vi "climbLoop.vi"() -> ()   [LabVIEW 2018]
uses:
  climbSMEnum.ctl
  climbStateEnum.ctl
  climbPlatformEnum.ctl
  climbStilt/climbStiltStateEnum.ctl
  driveClimbStateEnum.ctl
  <userlib>/836-Library/System/TDMS_V2/Support/TDMS_DevRef.ctl
  <userlib>/836-Library/System/TDMS_V2/Support/Logging_Settings.ctl
  <userlib>/836-Library/System/TDMS_V2/Support/Group_FIFO_Config.ctl
  <userlib>/836-Library/System/TDMS_V2/Support/Channel_FIFO_Config.ctl
panel:
  in  "Drive Enc Trig Point L2":dbl=-35.0
  out "timed out?":bool=TRUE
  in  "Drive Enc Trig Point L3":dbl=-35.0
  in  "Drive Speed":dbl=-0.2
  in  "Encoder Trigger Point":dbl=-12.9
  out "Waveform Chart":u16(graph)=12
  out "driveAvgPos(inch)":dbl=-5.765416124131944
  in  "Little wheel abs Power First 2":dbl=0.9
  in  "Wait to Extend (ms)":u32=500
  in  "Little wheel abs Power First":dbl=0.6
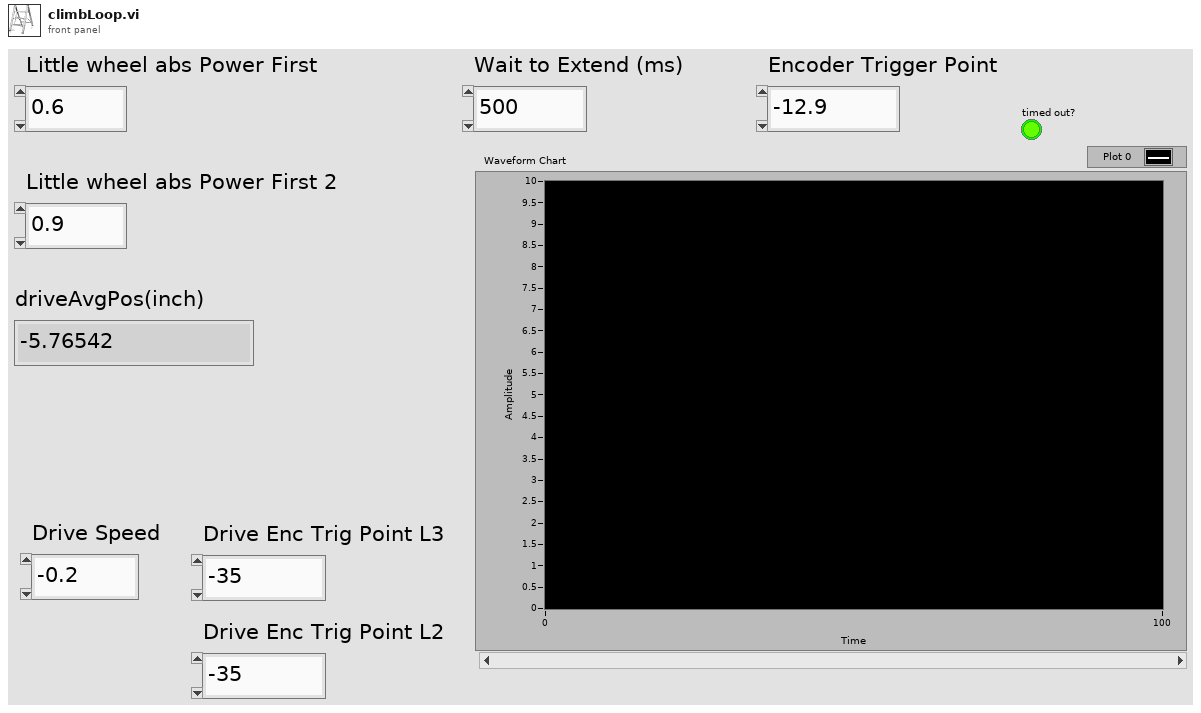
[diagram p1: front panel]
types:
  T1 = typedef "climbStateEnum.ctl" = enum16{"doNothing", "Auto Mode", "Safely Lower", "Test Mode"}
  T2 = typedef "climbSMEnum.ctl" = enum16{"1 - do nothing", "2 - Prep Systems", "3 - small startz", "4 - lift stiltz", "5 - drive little wheel 1", "6 - retract front stilt", "7 - drive little wheel 2", "8 - retract rear stilt", "9 - drive to middle", "10 - STOP", "7b - L2-L3 Drive Little Wheel 2", "8b - Balance", "10b - Balance Drive"}
  T3 = typedef "WPI_MotorControlDeviceRef.ctl" = cluster{"DeviceStatus":errorcluster, "Type":T4, "PWM":cluster{"PWM Channel":T5, "DeadBand":T6}, "CAN":cluster{"Device Number":u8, "SetOutput VI Ref":variant, "GetOutput VI Ref":variant, "Enable VI Ref":variant, "Disable VI Ref":variant, "Data":variant}, "Invert":bool, "DIO PWM":cluster{"PWM \"Enable\" Channel":T5, "DIOChannel":T7, "PWM Rate":dbl}}
  T4 = typedef "WPI_MotorControlType.ctl" = enum16{"PWM", "CAN", "DIO PWM"}
  T5 = typedef "FPGA_DIOPWMChannel.ctl" = enum8{"PWM 0", "PWM 1", "PWM 2", "PWM 3", "PWM 4", "PWM 5", "PWM 6", "PWM 7", "PWM 8", "PWM 9", "PWM MXP 0", "PWM MXP 1", "PWM MXP 2", "PWM MXP 3", "PWM MXP 4", "PWM MXP 5", "PWM MXP 6", "PWM MXP 7", "PWM MXP 8", "PWM MXP 9", "Invalid"}
  T6 = typedef "WPI_PWMDeadband.ctl" = cluster{"Name":string, "maxPositivePwm":i32, "minPositivePwm":i32, "centerPwm":i32, "maxNegativePwm":i32, "minNegativePwm":i32, "angularRange":u16}
  T7 = typedef "FPGA_DIOChannel.ctl" = enum8{"DIO 0", "DIO 1", "DIO 2", "DIO 3", "DIO 4", "DIO 5", "DIO 6", "DIO 7", "DIO 8", "DIO 9", "DIO MXP 0", "DIO MXP 1", "DIO MXP 2", "DIO MXP 3", "DIO MXP 4", "DIO MXP 5", "DIO MXP 6", "DIO MXP 7", "DIO MXP 8", "DIO MXP 9", "DIO MXP 10", "DIO MXP 11", "DIO MXP 12", "DIO MXP 13", "DIO MXP 14", "DIO MXP 15", "SPI Port CS1", "SPI Port CS2", "SPI Port CS3", "SPI Port MISO", "SPI Port MOSI", "Invalid"}
  T8 = typedef "WPI_DigitalInputDevRef.ctl" = cluster{"DevStatus":errorcluster, "DIO Channel":T7}
  T9 = typedef "WPI_SolenoidDevRef.ctl" = cluster{"DevStatus":errorcluster, "Pneumatics Control Module":u8, "Forward Solenoid Channel":T10, "Reverse Solenoid Channel":T10}
  T10 = typedef "WPI_SolenoidChannel.ctl" = enum8{"Solenoid 0", "Solenoid 1", "Solenoid 2", "Solenoid 3", "Solenoid 4", "Solenoid 5", "Solenoid 6", "Solenoid 7", "Invalid"}
  T11 = enum16{"L1 -> L3 Platform", "L1 -> L2 Platform", "L2 -> L3 Platform", "No Climb"}
  T12 = enum16{"Both Locked", "Skid Unlock/Powered Locked", "Skid Locked/Powered Unlocked", "Both Unlocked"}
  T13 = typedef "climbPlatformEnum.ctl" = enum16{"L1 -> L3 Platform", "L1 -> L2 Platform", "L2 -> L3 Platform", "No Climb"}
  T14 = typedef "driveClimbStateEnum.ctl" = enum16{"Do Nothing", "Drive Forward", "Slow Manual Drive"}
  T15 = typedef "climbStiltStateEnum.ctl" = enum16{"doNothing", "Start/Safely Lower Both", "Both Extend", "Front Retract", "Both Retract", "Test Mode", "Balance"}
  T16 = typedef "TDMS_DevRef.ctl" = cluster{"Name":string, "File Ref":refnum<k34>, "Start Time":timestamp, "Logging Settings":T17, "Group FIFO Config":T18[], "Data To Write":refnum<data-value>, "semaphore":T20, "Ref Time Reset":refnum<k4>}
  T17 = typedef "Logging_Settings.ctl" = cluster{"Data Grab Period":dbl, "File Write Period":dbl, "Max Stored Size":dbl, "Burst Size":dbl}
  T18 = typedef "Group_FIFO_Config.ctl" = cluster{"Group":string, "Channels":T19[], "Channel Names":string[]}
  T19 = typedef "Channel_FIFO_Config.ctl" = cluster{"Channel":string, "FIFO":refnum<k33>}
  T20 = typedef "Semaphore RefNum" = refnum<k1>
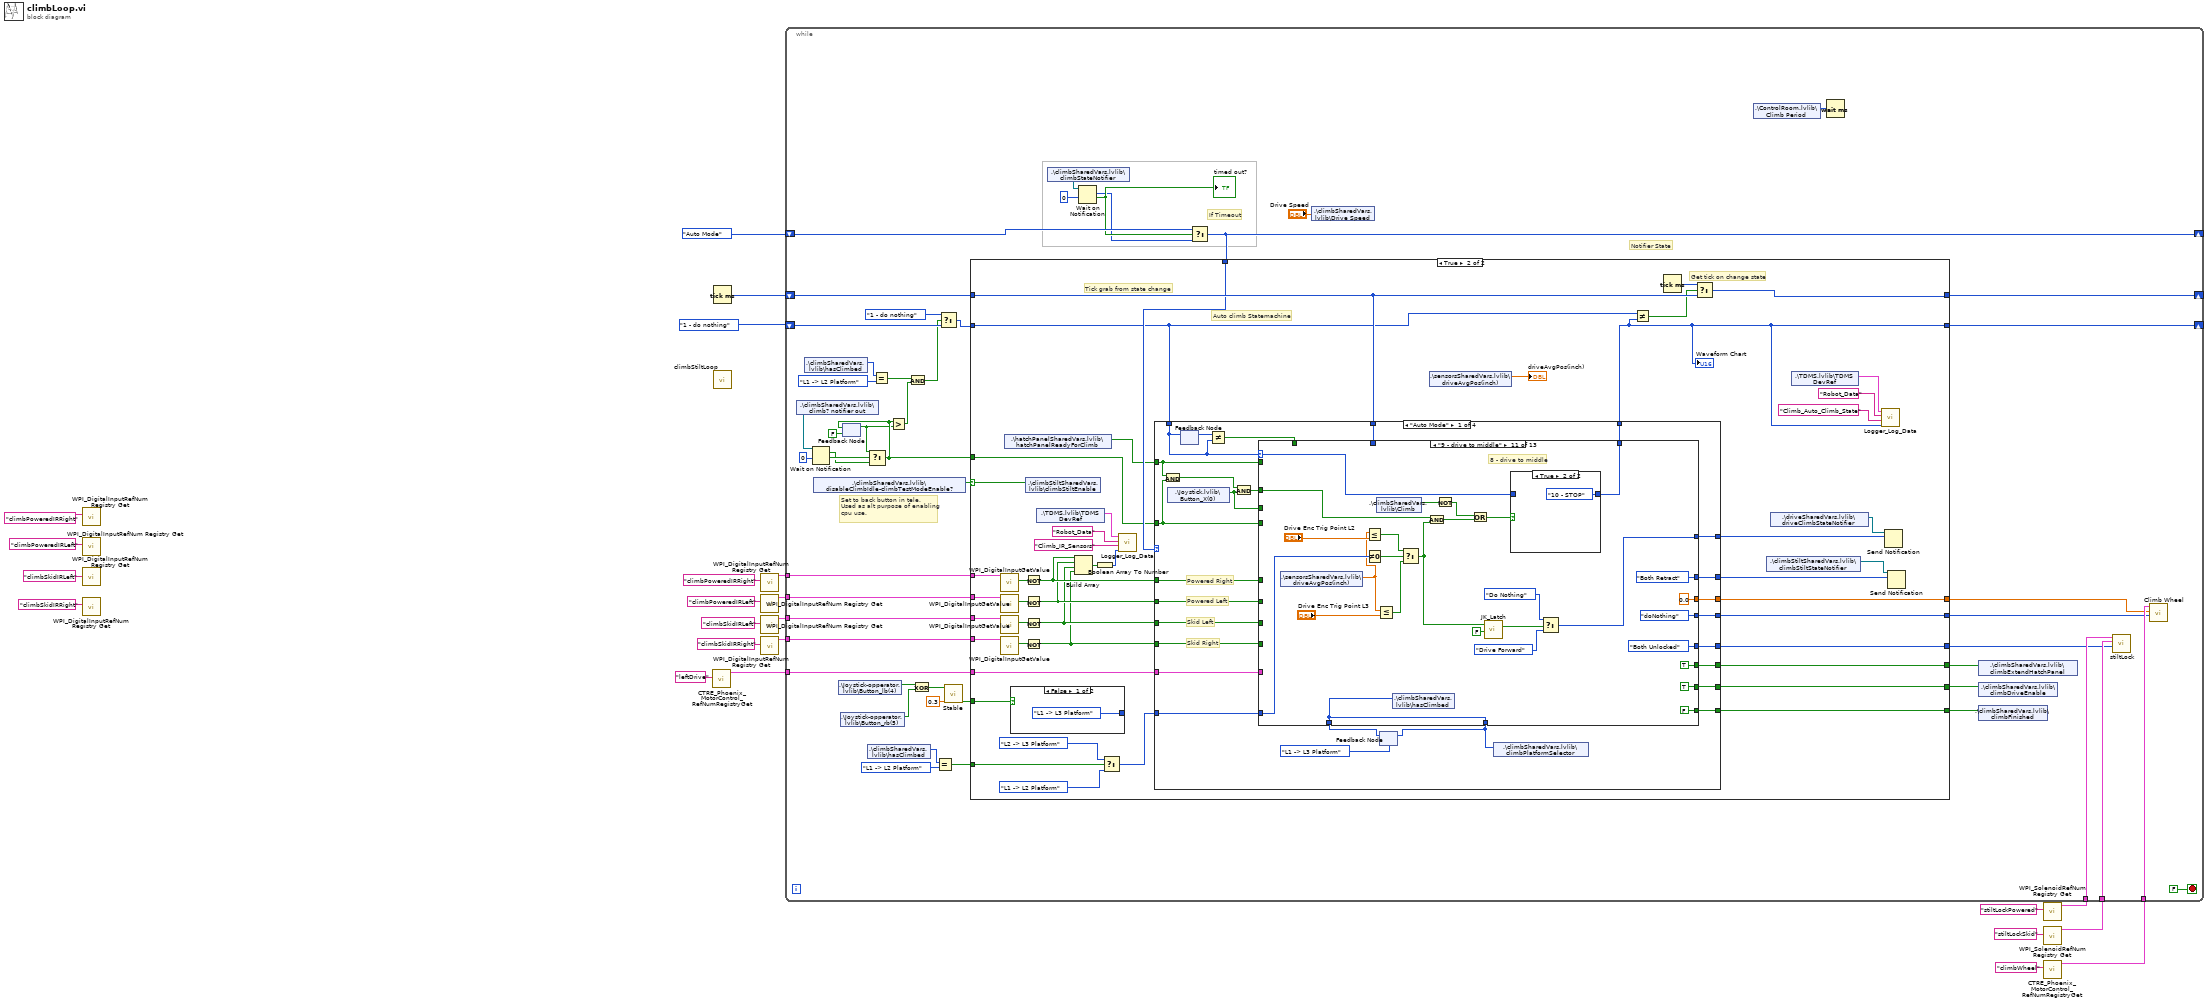
[diagram p0: block diagram]
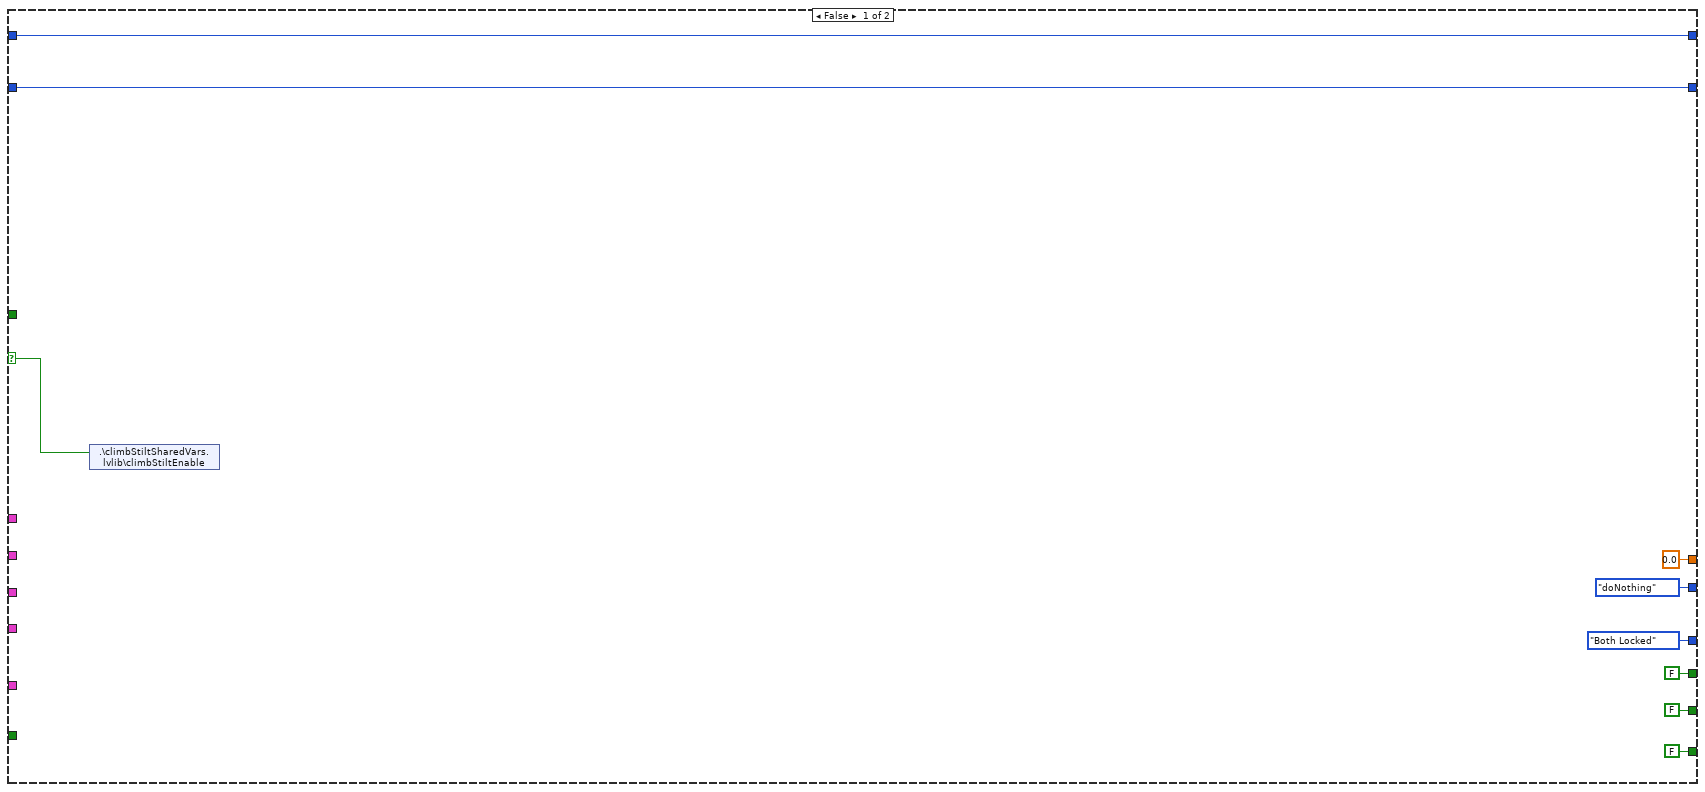
[diagram p2: hidden frame]
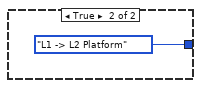
[diagram p3: hidden frame]
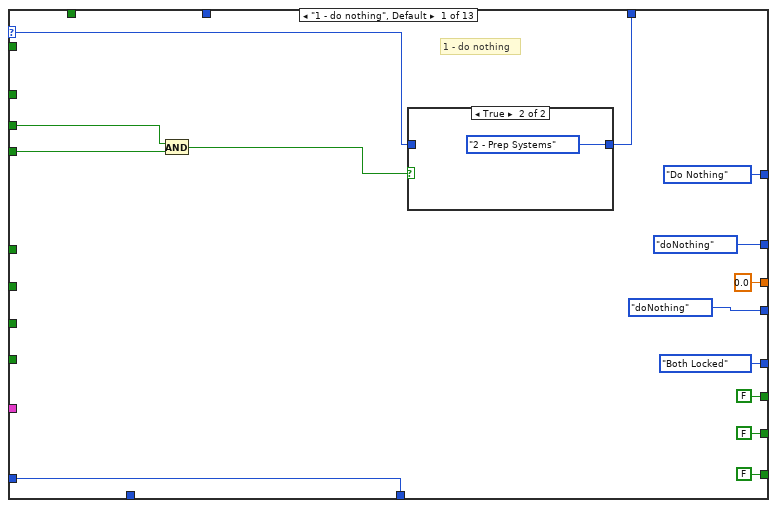
[diagram p4: hidden frame]
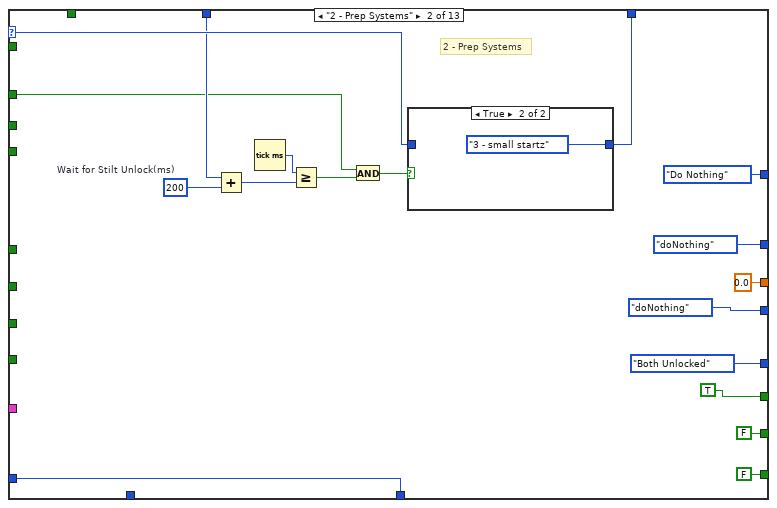
[diagram p6: hidden frame]
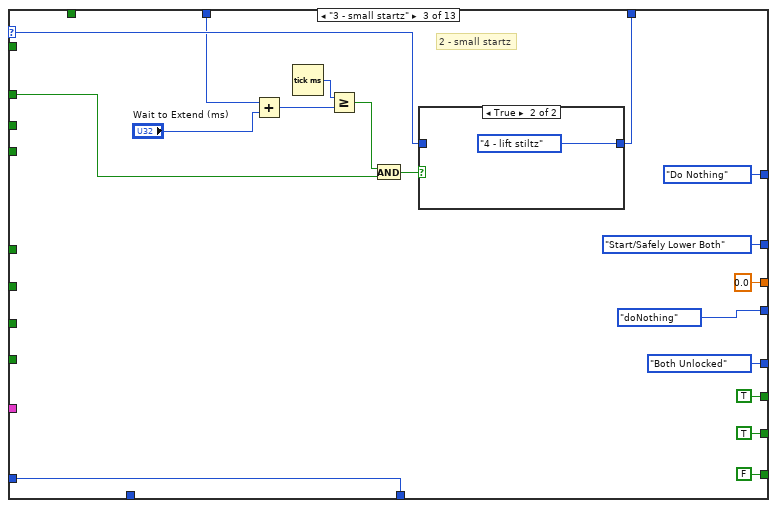
[diagram p8: hidden frame]
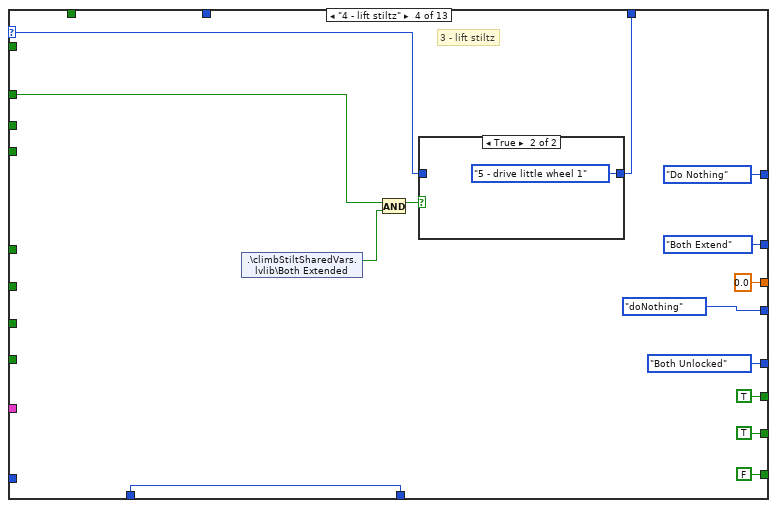
[diagram p10: hidden frame]
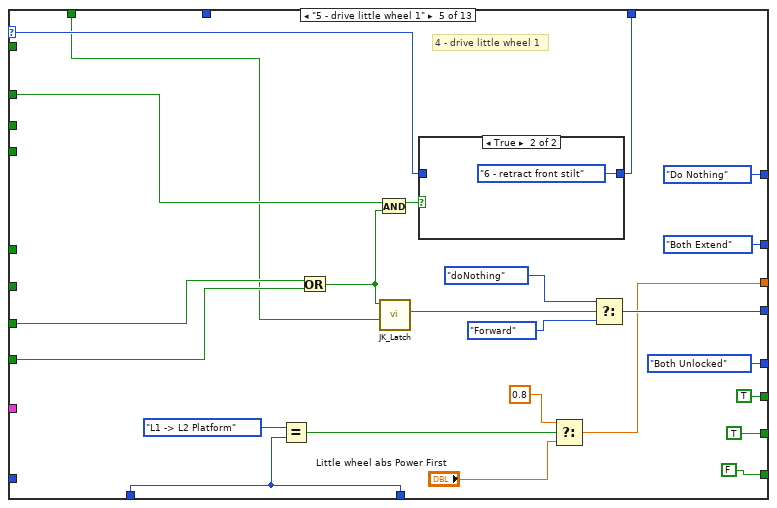
[diagram p12: hidden frame]
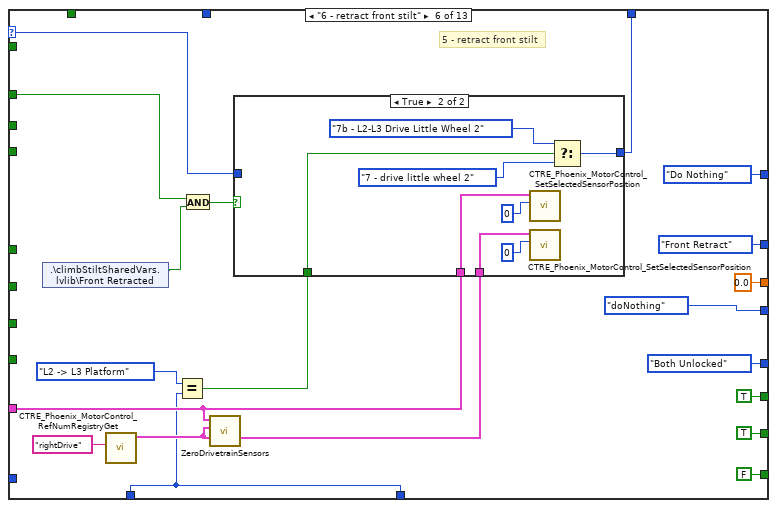
[diagram p14: hidden frame]
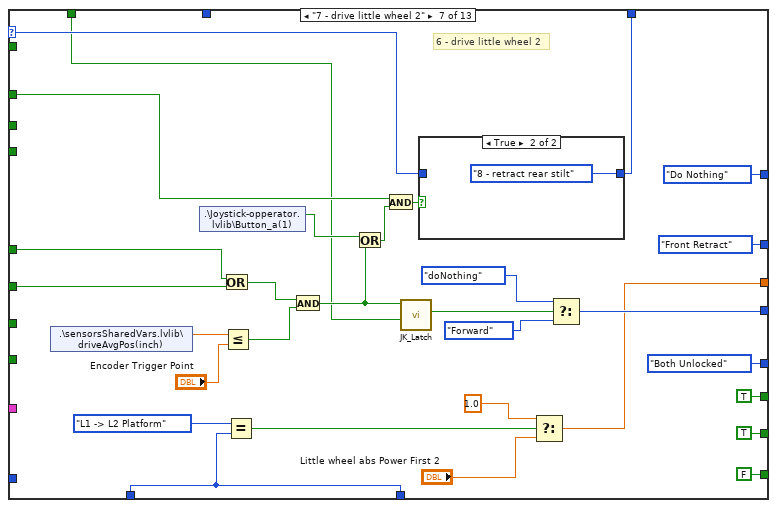
[diagram p16: hidden frame]
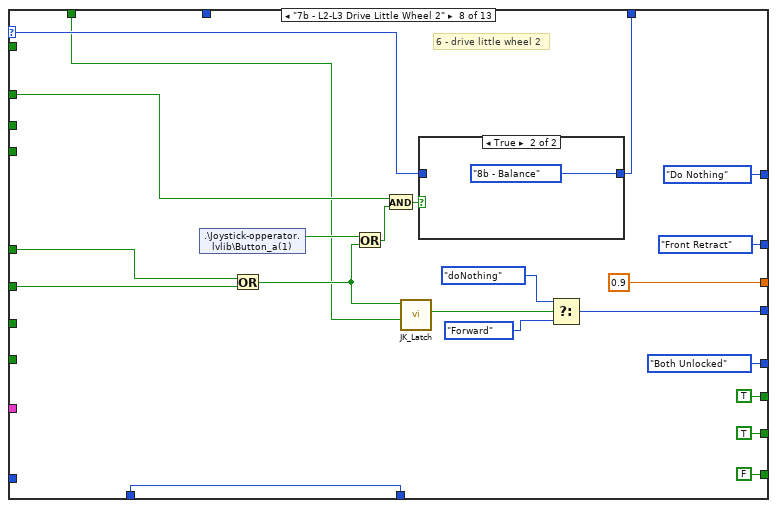
[diagram p18: hidden frame]
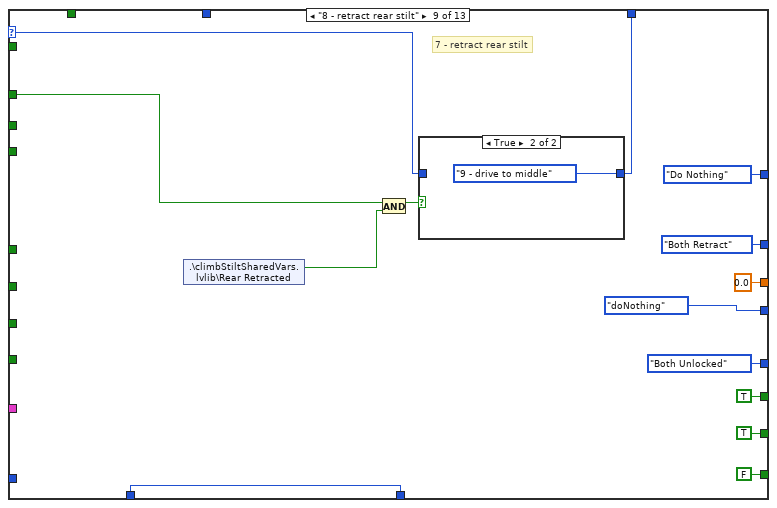
[diagram p20: hidden frame]
diagram:
  n1 = call <vilib>:"WPI_DigitalInputRefNum Registry Get.vi"("refnum name"="climbPoweredIRRight") -> ()  [unwired: 9 in, 2 out]
  n2 = call <vilib>:"WPI_DigitalInputRefNum Registry Get.vi"("refnum name"="climbPoweredIRLeft") -> ()  [unwired: 9 in, 2 out]
  n3 = call <vilib>:"WPI_DigitalInputRefNum Registry Get.vi"("refnum name"="climbSkidIRLeft") -> ()  [unwired: 9 in, 2 out]
  n4 = call <vilib>:"WPI_DigitalInputRefNum Registry Get.vi"("refnum name"="climbSkidIRRight") -> ()  [unwired: 9 in, 2 out]
  n5 = call <vilib>:"CTRE_Phoenix_MotorControl_RefNumRegistryGet.vi"("refnum name"="leftDrive") -> ("PhoenixMotorControlDevRef"=w21:T3)  [unwired: 9 in, 1 out]
  n6 = Tick Count (ms)() -> (millisecond timer value=w23:u32)
  n7 = call "climbStiltLoop.vi"() -> ()  [unwired: 12 in]
  n8 = call <vilib>:"WPI_DigitalInputRefNum Registry Get.vi"("refnum name"="climbPoweredIRRight") -> ("DigitalInputDevRef"=w1:T8)  [unwired: 9 in, 1 out]
  n9 = call <vilib>:"WPI_DigitalInputRefNum Registry Get.vi"("refnum name"="climbPoweredIRLeft") -> ("DigitalInputDevRef"=w2:T8)  [unwired: 9 in, 1 out]
  n10 = call <vilib>:"WPI_DigitalInputRefNum Registry Get.vi"("refnum name"="climbSkidIRLeft") -> ("DigitalInputDevRef"=w3:T8)  [unwired: 9 in, 1 out]
  n11 = call <vilib>:"WPI_DigitalInputRefNum Registry Get.vi"("refnum name"="climbSkidIRRight") -> ("DigitalInputDevRef"=w4:T8)  [unwired: 9 in, 1 out]
  n12 = call <vilib>:"WPI_SolenoidRefNum Registry Get.vi"("refnum name"="stiltLockPowered") -> ("SolenoidDevRef"=w18:T9)  [unwired: 9 in, 1 out]
  n13 = call <vilib>:"WPI_SolenoidRefNum Registry Get.vi"("refnum name"="stiltLockSkid") -> ("SolenoidDevRef"=w17:T9)  [unwired: 9 in, 1 out]
  n14 = call <vilib>:"CTRE_Phoenix_MotorControl_RefNumRegistryGet.vi"("refnum name"="climbWheel") -> ("PhoenixMotorControlDevRef"=w14:T3)  [unwired: 9 in, 1 out]
  n15 = while {
    shift-right: [w70] -> _
    shift-left: climbStateEnum."Auto Mode" ("Climb State") -> [w68]
    shift-right: [w69] -> _
    shift-left: climbSMEnum."1 - do nothing" ("Climb SM") -> [w29]
    shift-right: [w73] -> _
    shift-left: w23 -> [w72]
    tunnel: w21 -> [w71]
    tunnel: w18 -> [w67]
    tunnel: w17 -> [w66]
    tunnel: w14 -> [w65]
    tunnel: w4 -> [w42]
    tunnel: w3 -> [w41]
    tunnel: w2 -> [w40]
    tunnel: w1 -> [w39]
    stop <- FALSE stop-if-true
    # "Set to back button in tele.\nUsed as alt purpose of enabling\ncpu use."
    # "Notifier State"
    # "If Timeout"
    n16 = shared-variable ".\\climbSharedVars.lvlib\\climb? notifier out"() -> (w51:refnum<notifier>)  [unwired: 1 in, 1 out]
    n17 = shared-variable ".\\climbSharedVars.lvlib\\hasClimbed"() -> (w36:T11)  [unwired: 1 in, 1 out]
    n18 = Wait on Notification(notifier=w51, timeout in ms (-1)=0) -> (notification=w52:bool, timed out?=w53:bool)  [unwired: 2 in, 2 out]
    n19 = shared-variable ".\\climbSharedVars.lvlib\\disableClimbIdle-climbTestModeEnable?"() -> (w48:bool)  [unwired: 1 in, 1 out]
    n20 = shared-variable ".\\Joystick-opperator.lvlib\\Button_lb(4)"() -> (w47:bool)  [unwired: 1 in, 1 out]
    n21 = shared-variable ".\\Joystick-opperator.lvlib\\Button_rb(5)"() -> (w46:bool)  [unwired: 1 in, 1 out]
    n22 = feedback #1(FALSE ("create if not found? (T)")) -> (w33:bool)
    n23 = shared-variable ".\\climbSharedVars.lvlib\\hasClimbed"() -> (w26:T11)  [unwired: 1 in, 1 out]
    n24 = Select(t=w33, s=w53, f=w52) -> (s? t:f=w34:bool)
    n25 = feedback-in #1(w34) -> ()
    n26 = Equal?(x=w36, y=T11."L1 -> L2 Platform") -> (x = y?=w31:bool)
    n27 = Greater?(x=w34, y=w33) -> (0:w32:bool)
    n28 = And(x=w31, y=w32) -> (x .and. y?=w28:bool)
    n29 = Exclusive Or(1:w46, 2:w47) -> (0:w45:bool)
    n30 = Equal?(x=w26, y=T11."L1 -> L2 Platform") -> (x = y?=w24:bool)
    n31 = Select(t=climbSMEnum."1 - do nothing", s=w28, f=w29) -> (s? t:f=w27:T2)
    n32 = call <userlib>:"Stable.vi"("Eval Period (sec)"=0.3, "Signal Input"=w45) -> ("Stable"=w44:bool)  [unwired: 9 in]
    n33 = shared-variable ".\\climbSharedVars.lvlib\\climbStateNotifier"() -> (w61:refnum<notifier>)  [unwired: 1 in, 1 out]
    n34 = Wait on Notification(notifier=w61, timeout in ms (-1)=0) -> (notification=w58:T1, timed out?=w62:bool)  [unwired: 2 in, 2 out]
    "timed out?" <- w62
    n35 = Select(t=w68, s=w62, f=w58) -> (s? t:f=w70:T1)
    n36 = case shown="True" w48 {
      selector: w48 -> [w75 w109]
      tunnel: [w76 w129] -> w73
      tunnel: w72 -> [w76 w128]
      tunnel: w71 -> [_ w127]
      tunnel: w70 -> [_ w126]
      tunnel: [w74 w125] -> w69
      tunnel: [enum16{"doNothing", "Forward", "Backward"}."doNothing" ("Enum") w124] -> w64
      tunnel: [0.0 ("Little wheel abs Power First 2") w119] -> w60
      tunnel: [FALSE w114] -> w57
      tunnel: [FALSE w113] -> w56
      tunnel: [FALSE w112] -> w55
      tunnel: [T12."Both Locked" ("Lock State") w111] -> w54
      tunnel: w34 -> [_ w110]
      tunnel: w44 -> [_ w105]
      tunnel: w42 -> [_ w100]
      tunnel: w41 -> [_ w99]
      tunnel: w40 -> [_ w98]
      tunnel: w39 -> [_ w97]
      tunnel: w27 -> [w74 w87]
      tunnel: w24 -> [_ w83]
      frame False {
        n37 = shared-variable ".\\climbStiltSharedVars.lvlib\\climbStiltEnable"(w75) -> ()  [unwired: 1 in, 1 out]
      }
      frame True {
        # "Auto climb Statemachine"
        # "Tick grab from state change"
        # "Get tick on change state"
        n38 = call <vilib>:"WPI_DigitalInputGetValue.vi"("DigitalInputDevRef"=w97) -> ("Value"=w101:bool)  [unwired: 8 in, 2 out]
        n39 = call <vilib>:"WPI_DigitalInputGetValue.vi"("DigitalInputDevRef"=w98) -> ("Value"=w102:bool)  [unwired: 8 in, 2 out]
        n40 = call <vilib>:"WPI_DigitalInputGetValue.vi"("DigitalInputDevRef"=w99) -> ("Value"=w103:bool)  [unwired: 8 in, 2 out]
        n41 = call <vilib>:"WPI_DigitalInputGetValue.vi"("DigitalInputDevRef"=w100) -> ("Value"=w104:bool)  [unwired: 8 in, 2 out]
        n42 = shared-variable ".\\hatchPanelSharedVars.lvlib\\hatchPanelReadyForClimb"() -> (w115:bool)  [unwired: 1 in, 1 out]
        n43 = case shown="False" w105 {
          tunnel: [climbPlatformEnum."L1 -> L3 Platform" ("climbPlatformSelector") climbPlatformEnum."L1 -> L2 Platform" ("climbPlatformSelector")] -> _
          frame False {
          }
          frame True {
          }
        }
        n44 = Not(x=w101) -> (.not. x?=w91:bool)
        n45 = Not(x=w102) -> (.not. x?=w90:bool)
        n46 = Not(x=w103) -> (.not. x?=w89:bool)
        n47 = Not(x=w104) -> (.not. x?=w88:bool)
        n48 = shared-variable ".\\climbStiltSharedVars.lvlib\\climbStiltEnable"(w109) -> ()  [unwired: 1 in, 1 out]
        n49 = shared-variable ".\\TDMS.lvlib\\TDMS DevRef"() -> (w95:T16)  [unwired: 1 in, 1 out]
        n50 = Build Array(w91, w90, w89, w88) -> (w92:bool[])
        n51 = Boolean Array To Number(Boolean array=w92) -> (number=w96:u32)
        n52 = Select(t=climbPlatformEnum."L2 -> L3 Platform" ("climbPlatformSelector"), s=w83, f=climbPlatformEnum."L1 -> L2 Platform" ("climbPlatformSelector")) -> (s? t:f=w85:T13)
        n53 = call <userlib>:"Logger_Log_Data.vi"("Data"=w96, "Channel"="Climb_IR_Sensors", "Group"="Robot_Data", "TDMS DevRef"=w95) -> ()  [unwired: 7 in, 1 out]
        n54 = case shown="\"Auto Mode\"" w126 {
          tunnel: [w158 enum16{"doNothing", "Forward", "Backward"}."doNothing" ("Enum") enum16{"doNothing", "Forward", "Backward"}."doNothing" ("Enum") enum16{"doNothing", "Forward", "Backward"}."doNothing" ("Enum")] -> w124
          tunnel: w87 -> [w133 _ _ _]
          tunnel: [w157 climbStiltStateEnum."Start/Safely Lower Both" ("notification") w440 climbStiltStateEnum."doNothing" ("notification")] -> w122
          tunnel: [w156 climbSMEnum."1 - do nothing" ("Climb SM") climbSMEnum."1 - do nothing" ("Climb SM") climbSMEnum."1 - do nothing" ("Climb SM")] -> w125
          tunnel: w128 -> [w155 _ _ _]
          tunnel: [w154 0.0 ("Little wheel abs Power First 2") 0.0 ("Little wheel abs Power First 2") 0.0 ("Little wheel abs Power First 2")] -> w119
          tunnel: w127 -> [w153 _ _ _]
          tunnel: [w152 driveClimbStateEnum."Do Nothing" ("notification") driveClimbStateEnum."Do Nothing" ("notification") driveClimbStateEnum."Do Nothing" ("notification")] -> w116
          tunnel: w110 -> [w148 _ _ _]
          tunnel: [w151 T12."Both Unlocked" ("Lock State") T12."Both Unlocked" ("Lock State") T12."Both Locked" ("Lock State")] -> w111
          tunnel: [w150 TRUE TRUE FALSE] -> w113
          tunnel: w115 -> [w149 _ w437 _]
          tunnel: [w147 TRUE TRUE FALSE] -> w114
          tunnel: [w146 FALSE FALSE FALSE] -> w112
          tunnel: w85 -> [w145 _ _ _]
          tunnel: w88 -> [w141 _ _ _]
          tunnel: w89 -> [w140 _ _ _]
          tunnel: w90 -> [w139 _ _ _]
          tunnel: w91 -> [w138 _ _ _]
          frame "Auto Mode" {
            # "Skid Right"
            # "Skid Left"
            # "Powered Left"
            # "Powered Right"
            n55 = And(x=w149, y=w148) -> (x .and. y?=w137:bool)
            n56 = shared-variable ".\\Joystick.lvlib\\Button_X(0)"() -> (w135:bool)  [unwired: 1 in, 1 out]
            n57 = feedback-in #2(w133) -> ()
            n58 = feedback #2() -> (w134:T2)  [unwired: 1 in]
            n59 = Not Equal?(x=w134, y=w133) -> (x != y?=w132:bool)
            n60 = And(x=w137, y=w135) -> (x .and. y?=w136:bool)
            n61 = feedback #3(climbPlatformEnum."L1 -> L3 Platform" ("climbPlatformSelector")) -> (w143:T13)
            n62 = case shown="\"9 - drive to middle\"" w133 {
              selector: w133 -> [w169 w189 w209 w228 w254 w275 w314 w338 w354 w374 w394 w414 w424]
              tunnel: [enum16{"doNothing", "Forward", "Backward"}."doNothing" ("Enum") enum16{"doNothing", "Forward", "Backward"}."doNothing" ("Enum") enum16{"doNothing", "Forward", "Backward"}."doNothing" ("Enum") enum16{"doNothing", "Forward", "Backward"}."doNothing" ("Enum") w248 enum16{"doNothing", "Forward", "Backward"}."doNothing" ("Enum") w309 w333 enum16{"doNothing", "Forward", "Backward"}."doNothing" ("Enum") enum16{"doNothing", "Forward", "Backward"}."doNothing" ("Enum") enum16{"doNothing", "Forward", "Backward"}."doNothing" ("Enum") enum16{"doNothing", "Forward", "Backward"}."doNothing" ("Enum") enum16{"doNothing", "Forward", "Backward"}."doNothing" ("Enum")] -> w158
              tunnel: [climbStiltStateEnum."doNothing" ("notification") climbStiltStateEnum."doNothing" ("notification") climbStiltStateEnum."Start/Safely Lower Both" ("notification") climbStiltStateEnum."Both Extend" ("notification") climbStiltStateEnum."Both Extend" ("notification") climbStiltStateEnum."Front Retract" ("notification") climbStiltStateEnum."Front Retract" ("notification") climbStiltStateEnum."Front Retract" ("notification") climbStiltStateEnum."Both Retract" ("notification") climbStiltStateEnum."Balance" ("notification") climbStiltStateEnum."Both Retract" ("notification") climbStiltStateEnum."doNothing" ("notification") climbStiltStateEnum."doNothing" ("notification")] -> w157
              tunnel: [w170 w190 w210 w227 w253 w274 w313 w337 w353 w373 w393 w414 w424] -> w156
              tunnel: w155 -> [_ w180 w204 _ _ _ _ _ _ w357 _ _ _]
              tunnel: [0.0 ("Little wheel abs Power First 2") 0.0 ("Little wheel abs Power First 2") 0.0 ("Little wheel abs Power First 2") 0.0 ("Little wheel abs Power First 2") w236 0.0 ("Little wheel abs Power First 2") w290 0.9 ("t") 0.0 ("Little wheel abs Power First 2") 0.0 ("Little wheel abs Power First 2") 0.0 ("Little wheel abs Power First 2") 0.0 ("Little wheel abs Power First 2") 0.0 ("Little wheel abs Power First 2")] -> w154
              tunnel: w153 -> [_ _ _ _ _ w262 _ _ _ _ _ _ _]
              tunnel: [driveClimbStateEnum."Do Nothing" ("notification") driveClimbStateEnum."Do Nothing" ("notification") driveClimbStateEnum."Do Nothing" ("notification") driveClimbStateEnum."Do Nothing" ("notification") driveClimbStateEnum."Do Nothing" ("notification") driveClimbStateEnum."Do Nothing" ("notification") driveClimbStateEnum."Do Nothing" ("notification") driveClimbStateEnum."Do Nothing" ("notification") driveClimbStateEnum."Do Nothing" ("notification") driveClimbStateEnum."Do Nothing" ("notification") w398 driveClimbStateEnum."Do Nothing" ("notification") driveClimbStateEnum."Slow Manual Drive" ("notification")] -> w152
              tunnel: w136 -> [_ w177 w200 w220 w245 w267 w302 w329 w346 w359 w392 _ _]
              tunnel: w145 -> [w162 w175 w195 _ _ _ _ _ _ _ w391 _ _]
              tunnel: [T12."Both Locked" ("Lock State") T12."Both Unlocked" ("Lock State") T12."Both Unlocked" ("Lock State") T12."Both Unlocked" ("Lock State") T12."Both Unlocked" ("Lock State") T12."Both Unlocked" ("Lock State") T12."Both Unlocked" ("Lock State") T12."Both Unlocked" ("Lock State") T12."Both Unlocked" ("Lock State") T12."Both Unlocked" ("Lock State") T12."Both Unlocked" ("Lock State") T12."Both Locked" ("Lock State") T12."Both Locked" ("Lock State")] -> w151
              tunnel: [FALSE TRUE TRUE TRUE TRUE TRUE TRUE TRUE TRUE TRUE TRUE TRUE TRUE] -> w150
              tunnel: w149 -> [_ _ _ _ _ _ _ _ _ _ _ _ _]
              tunnel: w148 -> [w161 _ _ _ _ _ _ _ _ _ _ _ _]
              tunnel: [FALSE FALSE TRUE TRUE TRUE TRUE TRUE TRUE TRUE TRUE TRUE FALSE TRUE] -> w147
              tunnel: [FALSE FALSE FALSE FALSE FALSE FALSE FALSE FALSE FALSE FALSE FALSE TRUE TRUE] -> w146
              tunnel: [w162 w175 w195 w215 w233 w258 w289 w319 w341 w363 w380 w407 w417] -> w142
              tunnel: w143 -> [_ _ _ w215 w233 w258 w289 w319 w341 w363 w380 w407 w417]
              tunnel: w141 -> [_ _ _ _ w239 _ _ _ _ _ _ _ _]
              tunnel: w140 -> [_ _ _ _ w238 _ _ _ _ _ _ _ _]
              tunnel: w139 -> [_ _ _ _ _ _ w293 w321 _ _ _ _ _]
              tunnel: w138 -> [_ _ _ _ _ _ w292 w320 _ _ _ _ _]
              tunnel: w135 -> [w160 _ _ _ _ _ _ _ _ _ _ _ _]
              tunnel: w132 -> [_ _ _ _ w231 _ w285 w318 _ _ _ _ _]
              frame "1 - do nothing", Default {
                # "1 - do nothing"
                n63 = And(x=w160, y=w161) -> (x .and. y?=w159:bool)
                n64 = case shown="True" w159 {
                  tunnel: [w173 climbSMEnum."2 - Prep Systems" ("Climb SM")] -> w170
                  tunnel: w169 -> [w173 _]
                  frame False {
                  }
                  frame True {
                  }
                }
              }
              frame "2 - Prep Systems" {
                w179 = u32 200  # Wait for Stilt Unlock(ms)
                # "2 - Prep Systems"
                n65 = Add(x=w180, y=w179) -> (x+y=w181:u32)
                n66 = Tick Count (ms)() -> (millisecond timer value=w182:u32)
                n67 = Greater Or Equal?(x=w182, y=w181) -> (x >= y?=w176:bool)
                n68 = And(x=w177, y=w176) -> (x .and. y?=w178:bool)
                n69 = case shown="True" w178 {
                  tunnel: [w193 climbSMEnum."3 - small startz" ("Climb SM")] -> w190
                  tunnel: w189 -> [w193 _]
                  frame False {
                  }
                  frame True {
                  }
                }
              }
              frame "3 - small startz" {
                # "2 - small startz"
                n70 = Add(x=w204, y="Wait to Extend (ms)") -> (x+y=w205:u32)
                n71 = Tick Count (ms)() -> (millisecond timer value=w207:u32)
                n72 = Greater Or Equal?(x=w207, y=w205) -> (x >= y?=w206:bool)
                n73 = And(x=w206, y=w200) -> (x .and. y?=w208:bool)
                n74 = case shown="True" w208 {
                  tunnel: [w213 climbSMEnum."4 - lift stiltz" ("Climb SM")] -> w210
                  tunnel: w209 -> [w213 _]
                  frame False {
                  }
                  frame True {
                  }
                }
              }
              frame "4 - lift stiltz" {
                # "3 - lift stiltz"
                n75 = shared-variable ".\\climbStiltSharedVars.lvlib\\Both Extended"() -> (w223:bool)  [unwired: 1 in, 1 out]
                n76 = And(x=w220, y=w223) -> (x .and. y?=w224:bool)
                n77 = case shown="True" w224 {
                  tunnel: [w229 climbSMEnum."5 - drive little wheel 1" ("Climb SM")] -> w227
                  tunnel: w228 -> [w229 _]
                  frame False {
                  }
                  frame True {
                  }
                }
              }
              frame "5 - drive little wheel 1" {
                # "4 - drive little wheel 1"
                n78 = Equal?(x=climbPlatformEnum."L1 -> L2 Platform", y=w233) -> (x = y?=w234:bool)
                n79 = Or(x=w238, y=w239) -> (x .or. y?=w244:bool)
                n80 = And(x=w245, y=w244) -> (x .and. y?=w251:bool)
                n81 = call <userlib>:"JK_Latch.vi"("Reset"=w231, "Set"=w244) -> ("Q"=w247:bool)  [unwired: 5 in]
                n82 = case shown="True" w251 {
                  tunnel: [w255 climbSMEnum."6 - retract front stilt" ("Climb SM")] -> w253
                  tunnel: w254 -> [w255 _]
                  frame False {
                  }
                  frame True {
                  }
                }
                n83 = Select(t=0.8, s=w234, f="Little wheel abs Power First") -> (s? t:f=w236:dbl)
                n84 = Select(t=enum16{"doNothing", "Forward", "Backward"}."doNothing", s=w247, f=enum16{"doNothing", "Forward", "Backward"}."Forward" ("Enum")) -> (s? t:f=w248:enum16{"doNothing", "Forward", "Backward"})
              }
              frame "6 - retract front stilt" {
                # "5 - retract front stilt"
                n85 = shared-variable ".\\climbStiltSharedVars.lvlib\\Front Retracted"() -> (w270:bool)  [unwired: 1 in, 1 out]
                n86 = call <vilib>:"CTRE_Phoenix_MotorControl_RefNumRegistryGet.vi"("refnum name"="rightDrive") -> ("PhoenixMotorControlDevRef"=w260:T3)  [unwired: 9 in, 1 out]
                n87 = Equal?(x=climbPlatformEnum."L2 -> L3 Platform" ("climbPlatformSelector"), y=w258) -> (x = y?=w257:bool)
                n88 = And(x=w267, y=w270) -> (x .and. y?=w271:bool)
                n89 = call "ZeroDrivetrainSensors.vi"("Talon 2"=w260, "Talon 1"=w262) -> ()  [unwired: 8 in, 2 out]
                n90 = case shown="True" w271 {
                  tunnel: [w276 w280] -> w274
                  tunnel: w275 -> [w276 _]
                  tunnel: w262 -> [_ w283]
                  tunnel: w260 -> [_ w281]
                  tunnel: w257 -> [_ w277]
                  frame False {
                  }
                  frame True {
                    n91 = call <vilib>:"CTRE_Phoenix_MotorControl_SetSelectedSensorPosition.vi"("New Sensor Position"=0, "PhoenixMotorControlDevRef"=w283) -> ()  [unwired: 8 in, 2 out]
                    n92 = call <vilib>:"CTRE_Phoenix_MotorControl_SetSelectedSensorPosition.vi"("New Sensor Position"=0, "PhoenixMotorControlDevRef"=w281) -> ()  [unwired: 8 in, 2 out]
                    n93 = Select(t=climbSMEnum."7b - L2-L3 Drive Little Wheel 2" ("Climb SM"), s=w277, f=climbSMEnum."7 - drive little wheel 2" ("Climb SM")) -> (s? t:f=w280:T2)
                  }
                }
              }
              frame "7 - drive little wheel 2" {
                # "6 - drive little wheel 2"
                n94 = shared-variable ".\\sensorsSharedVars.lvlib\\driveAvgPos(inch)"() -> (w306:dbl)  [unwired: 1 in, 1 out]
                n95 = shared-variable ".\\Joystick-opperator.lvlib\\Button_a(1)"() -> (w294:bool)  [unwired: 1 in, 1 out]
                n96 = Or(x=w292, y=w293) -> (x .or. y?=w301:bool)
                n97 = Less Or Equal?(x=w306, y="Encoder Trigger Point") -> (x <= y?=w304:bool)
                n98 = Equal?(x=climbPlatformEnum."L1 -> L2 Platform", y=w289) -> (x = y?=w287:bool)
                n99 = And(x=w301, y=w304) -> (x .and. y?=w295:bool)
                n100 = Or(x=w294, y=w295) -> (x .or. y?=w296:bool)
                n101 = And(x=w302, y=w296) -> (x .and. y?=w310:bool)
                n102 = call <userlib>:"JK_Latch.vi"("Reset"=w285, "Set"=w295) -> ("Q"=w307:bool)  [unwired: 5 in]
                n103 = case shown="True" w310 {
                  tunnel: [w315 climbSMEnum."8 - retract rear stilt" ("Climb SM")] -> w313
                  tunnel: w314 -> [w315 _]
                  frame False {
                  }
                  frame True {
                  }
                }
                n104 = Select(t=1.0, s=w287, f="Little wheel abs Power First 2") -> (s? t:f=w290:dbl)
                n105 = Select(t=enum16{"doNothing", "Forward", "Backward"}."doNothing", s=w307, f=enum16{"doNothing", "Forward", "Backward"}."Forward" ("Enum")) -> (s? t:f=w309:enum16{"doNothing", "Forward", "Backward"})
              }
              frame "7b - L2-L3 Drive Little Wheel 2" {
                # "6 - drive little wheel 2"
                n106 = shared-variable ".\\Joystick-opperator.lvlib\\Button_a(1)"() -> (w322:bool)  [unwired: 1 in, 1 out]
                n107 = Or(x=w320, y=w321) -> (x .or. y?=w328:bool)
                n108 = Or(x=w322, y=w328) -> (x .or. y?=w323:bool)
                n109 = And(x=w329, y=w323) -> (x .and. y?=w334:bool)
                n110 = call <userlib>:"JK_Latch.vi"("Reset"=w318, "Set"=w328) -> ("Q"=w331:bool)  [unwired: 5 in]
                n111 = case shown="True" w334 {
                  tunnel: [w339 climbSMEnum."8b - Balance" ("Climb SM")] -> w337
                  tunnel: w338 -> [w339 _]
                  frame False {
                  }
                  frame True {
                  }
                }
                n112 = Select(t=enum16{"doNothing", "Forward", "Backward"}."doNothing", s=w331, f=enum16{"doNothing", "Forward", "Backward"}."Forward" ("Enum")) -> (s? t:f=w333:enum16{"doNothing", "Forward", "Backward"})
              }
              frame "8 - retract rear stilt" {
                # "7 - retract rear stilt"
                n113 = shared-variable ".\\climbStiltSharedVars.lvlib\\Rear Retracted"() -> (w349:bool)  [unwired: 1 in, 1 out]
                n114 = And(x=w346, y=w349) -> (x .and. y?=w350:bool)
                n115 = case shown="True" w350 {
                  tunnel: [w355 climbSMEnum."9 - drive to middle" ("Climb SM")] -> w353
                  tunnel: w354 -> [w355 _]
                  frame False {
                  }
                  frame True {
                  }
                }
              }
              frame "8b - Balance" {
                w360 = u32 200  # Wait for Stilt Unlock(ms)
                # "7 - retract rear stilt"
                n116 = Add(x=w357, y=w360) -> (x+y=w361:u32)
                n117 = Tick Count (ms)() -> (millisecond timer value=w362:u32)
                n118 = Greater Or Equal?(x=w362, y=w361) -> (x >= y?=w358:bool)
                n119 = And(x=w358, y=w359) -> (x .and. y?=w370:bool)
                n120 = case shown="True" w370 {
                  tunnel: [w375 climbSMEnum."10b - Balance Drive" ("Climb SM")] -> w373
                  tunnel: w374 -> [w375 _]
                  frame False {
                  }
                  frame True {
                  }
                }
              }
              frame "9 - drive to middle" {
                # "8 - drive to middle"
                n121 = shared-variable ".\\sensorsSharedVars.lvlib\\driveAvgPos(inch)"() -> (w385:dbl)  [unwired: 1 in, 1 out]
                n122 = Less Or Equal?(x=w385, y="Drive Enc Trig Point L2") -> (x <= y?=w387:bool)
                n123 = Not Equal To 0?(x=w391) -> (x != 0?=w390:bool)
                n124 = shared-variable ".\\climbSharedVars.lvlib\\Climb"() -> (w378:bool)  [unwired: 1 in, 1 out]
                n125 = Less Or Equal?(x=w385, y="Drive Enc Trig Point L3") -> (x <= y?=w389:bool)
                n126 = shared-variable ".\\climbSharedVars.lvlib\\hasClimbed"(w380) -> ()  [unwired: 1 in, 1 out]
                n127 = Select(t=w387, s=w390, f=w389) -> (s? t:f=w388:bool)
                n128 = And(x=w392, y=w388) -> (x .and. y?=w395:bool)
                n129 = Not(x=w378) -> (.not. x?=w377:bool)
                n130 = Or(x=w377, y=w395) -> (x .or. y?=w379:bool)
                n131 = call <userlib>:"JK_Latch.vi"("Reset"=FALSE, "Set"=w388) -> ("Q"=w396:bool)  [unwired: 5 in]
                n132 = case shown="True" w379 {
                  tunnel: w394 -> [w405 _]
                  tunnel: [w405 climbSMEnum."10 - STOP" ("Climb SM")] -> w393
                  frame False {
                  }
                  frame True {
                  }
                }
                n133 = Select(t=driveClimbStateEnum."Do Nothing" ("notification"), s=w396, f=driveClimbStateEnum."Drive Forward" ("notification")) -> (s? t:f=w398:T14)
              }
              frame "10 - STOP" {
                # "9 - STOP"
                n134 = shared-variable ".\\climbSharedVars.lvlib\\hasClimbed"(w407) -> ()  [unwired: 1 in, 1 out]
              }
              frame "10b - Balance Drive" {
                # "9 - STOP"
                n135 = shared-variable ".\\climbSharedVars.lvlib\\hasClimbed"(w417) -> ()  [unwired: 1 in, 1 out]
              }
            }
            n136 = feedback-in #3(w142) -> ()
            n137 = shared-variable ".\\climbSharedVars.lvlib\\climbPlatformSelector"(w142) -> ()  [unwired: 1 in, 1 out]
          }
          frame "Safely Lower" {
          }
          frame "Test Mode" {
            n138 = shared-variable ".\\climbSharedVars.lvlib\\disableClimbIdle-climbTestModeEnable?"() -> (w438:bool)  [unwired: 1 in, 1 out]
            n139 = And(x=w437, y=w438) -> (x .and. y?=w441:bool)
            n140 = case shown="False" w441 {
              tunnel: [climbStiltStateEnum."doNothing" ("notification") climbStiltStateEnum."Test Mode" ("notification")] -> w440
              frame False {
              }
              frame True {
              }
            }
          }
          frame "doNothing", Default {
          }
        }
        "Waveform Chart" <- w125
        n141 = shared-variable ".\\sensorsSharedVars.lvlib\\driveAvgPos(inch)"() -> (→"driveAvgPos(inch)":dbl)  [unwired: 1 in, 1 out]
        n142 = Not Equal?(x=w87, y=w125) -> (x != y?=w120:bool)
        n143 = Tick Count (ms)() -> (millisecond timer value=w121:u32)
        n144 = Select(t=w121, s=w120, f=w128) -> (s? t:f=w129:u32)
        n145 = shared-variable ".\\climbStiltSharedVars.lvlib\\climbStiltStateNotifier"() -> (w123:refnum<notifier>)  [unwired: 1 in, 1 out]
        n146 = shared-variable ".\\driveSharedVars.lvlib\\driveClimbStateNotifier"() -> (w117:refnum<notifier>)  [unwired: 1 in, 1 out]
        n147 = shared-variable ".\\TDMS.lvlib\\TDMS DevRef"() -> (w107:T16)  [unwired: 1 in, 1 out]
        n148 = call <userlib>:"Logger_Log_Data.vi"("Data"=w125, "Channel"="Climb_Auto_Climb_State", "Group"="Robot_Data", "TDMS DevRef"=w107) -> ()  [unwired: 7 in, 1 out]
        n149 = Send Notification(notification=w116, notifier=w117) -> ()  [unwired: 1 in, 2 out]
        n150 = Send Notification(notification=w122, notifier=w123) -> ()  [unwired: 1 in, 2 out]
      }
    }
    n151 = shared-variable ".\\climbSharedVars.lvlib\\Drive Speed"("Drive Speed") -> ()  [unwired: 1 in, 1 out]
    n152 = shared-variable ".\\ControlRoom.lvlib\\Climb Period"() -> (w38:i64)  [unwired: 1 in, 1 out]
    n153 = Wait (ms)(milliseconds to wait=w38) -> ()  [unwired: 1 out]
    n154 = shared-variable ".\\climbSharedVars.lvlib\\climbExtendHatchPanel"(w56) -> ()  [unwired: 1 in, 1 out]
    n155 = shared-variable ".\\climbSharedVars.lvlib\\climbDriveEnable"(w57) -> ()  [unwired: 1 in, 1 out]
    n156 = shared-variable ".\\climbSharedVars.lvlib\\climbFinished"(w55) -> ()  [unwired: 1 in, 1 out]
    n157 = call "stiltLock.vi"("Powered Lock SolenoidDevRef"=w67, "Skid Lock SolenoidDevRef"=w66, "Lock State"=w54) -> ()  [unwired: 8 in]
    n158 = call "Climb Wheel.vi"("Enum"=w64, "Power"=w60, "PhoenixMotorControlDevRef"=w65) -> ()  [unwired: 9 in]
  }
